vi "Initialize Modules.vi"(8 "error in (no error)":errorcluster, 10 "Modules":refnum<class "Module.lvclass">[](array[class]), 11 "Initial Sequence in":refnum<class "Main Sequence.lvclass">) -> (0 "error out":errorcluster, 2 "Modules":refnum<class "Module.lvclass">[](array[class]), 3 "Initial Sequence out":refnum<class "Main Sequence.lvclass">)   [LabVIEW 2015, in "Main Sequence.lvclass"]
uses:
  Main Sequence.lvclass
  Module/Module/Module.lvclass
  Block Diagram/Init.Refs.ctl
  <vilib>/Utility/miscctls.llb/LVPointTypeDef.ctl
  Structures/Read Diagram.vi
  Structures/Read Location.vi
  Block Diagram/Block Diagram.lvclass
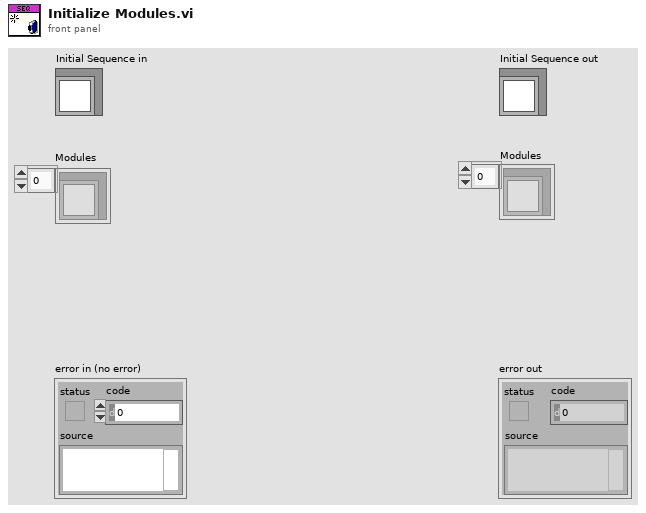
[diagram p1: front panel]
types:
  T1 = typedef "Block Diagram.lvclass/Init.Refs.ctl" = cluster{"Diagram":refnum<vi>, "Location":refnum<data-value>}
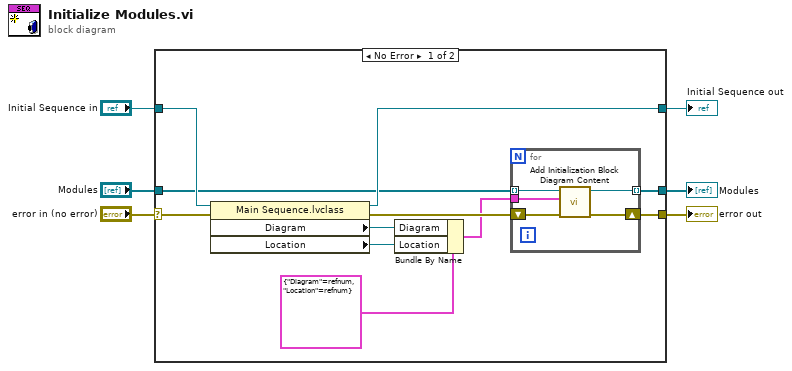
[diagram p0: block diagram]
diagram:
  n1 = case shown="No Error" "error in (no error)" {
    selector: "error in (no error)" -> [w17 w25]
    tunnel: [w12 w25] -> w5
    tunnel: [w15 w24] -> w3
    tunnel: "Initial Sequence in" -> [w16 w24]
    tunnel: "Modules" -> [w14 w23]
    tunnel: [w7 w23] -> w1
    frame No Error {
      n2 = property class="Main Sequence.lvclass"(reference=w16, error in=w17) -> (reference out=w15:refnum<class "Main Sequence.lvclass">, error out=w13:errorcluster, "Diagram"=w10:refnum<vi>, "Location"=w9:refnum<data-value>)
      n3 = Bundle By Name(cluster=T1 {"Diagram"=refnum, "Location"=refnum} ("Init"), "Diagram"=w10, "Location"=w9) -> (w8:T1)
      n4 = for {
        tunnel: w14 -> [w22] mode=indexing
        shift-right: [w20] -> w12
        shift-left: w13 -> [w21]
        tunnel: w8 -> [w19]
        tunnel: [w18] -> w7 mode=indexing
        n5 = call-dynamic "Add Initialization Block Diagram Content.vi"("error in (no error)"=w21, "Init"=w19, "Module in"=w22) -> ("error out"=w20:errorcluster, "Module out"=w18:refnum<class "Module.lvclass">)  [unwired: 7 in]
      }
    }
    frame Error {
    }
  }
  "error out" <- w5
  "Initial Sequence out" <- w3
  "Modules" <- w1
